vi "Load and Save Data (Bit Data).vi"(0 "VISA resource name":refnum<visa-resource-name>, 5 "Destination File":string, 7 "Data Block":string, 9 "Bit Count(0)":u32, 11 "error in (no error)":errorcluster) -> (4 "VISA resource name out":refnum<visa-resource-name>, 15 "error out":errorcluster)   [LabVIEW 2018, in "Agilent PSG MXG Series.lvlib"]
doc: "Loads bit data into signal generator memory and saves the data to a file.\n\n<B>Note:</B>\nThis VI is only valid in N5172B that installs with <B>Option 653</B> or <B>Option 655</B>, or N5182B that installs with <B>Option 656</B> or <B>Option 657</B>."
uses:
  Agilent PSG MXG Series.lvlib
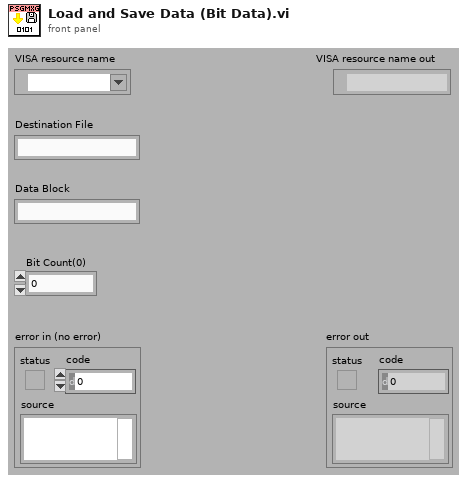
[diagram p1: front panel]
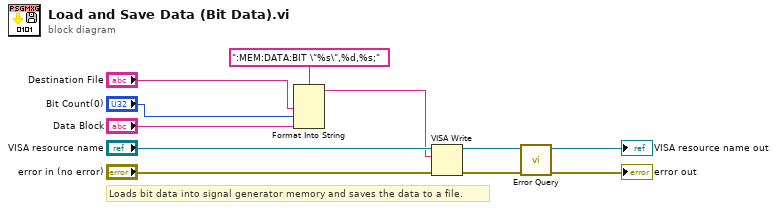
[diagram p0: block diagram]
diagram:
  # "Loads bit data into signal generator memory and saves the data to a file."
  n1 = Format Into String(format string=":MEM:DATA:BIT \"%s\",%d,%s;", "Destination File", "Bit Count(0)", "Data Block") -> (resulting string=w5:string)  [unwired: 2 in, 1 out]
  n2 = VISA Write(VISA resource name="VISA resource name", write buffer=w5, error in (no error)="error in (no error)") -> (VISA resource name out=w11:refnum<visa-resource-name>, error out=w10:errorcluster)  [unwired: 1 out]
  n3 = call "Error Query.vi"("error in (no error)"=w10, "VISA resource name"=w11) -> ("error out"=→"error out":errorcluster, "VISA resource name out"=→"VISA resource name out":refnum<visa-resource-name>)  [unwired: 6 in, 2 out]
